vi "tsc-Change Theme Edit--dialog.vi"(8 "error in":errorcluster, 11 "VI Refnum":refnum<vi>) -> (0 "error out":errorcluster)   [LabVIEW 2021]
doc: "Show this VI and let user define a new path/theme to apply to the VI.\n\n->Will be invoked with Quick Drop as a way to easily change the theme quickly during edit mode\n\n<b>Code Developed By:</b>\nTechnology Service Corporation\n1983 S Liberty Drive\nBloomington, IN 47403\nPhone: 812 558-7100\nwww.tsc.com/atcs\n\nDeveloper:\nDaniel Coons"
uses:
  Material Theme/Material Theme.lvclass
  user32.dll
panel:
  out "header":bool
  in  "Done":bool
  in  "Theme":u16(ring) items=["Light Theme", "Light Medium Contrast", "Light High Contrast", "Dark Theme", "Dark Medium Contrast", "Dark High Constrast"]
  in  "file path":path
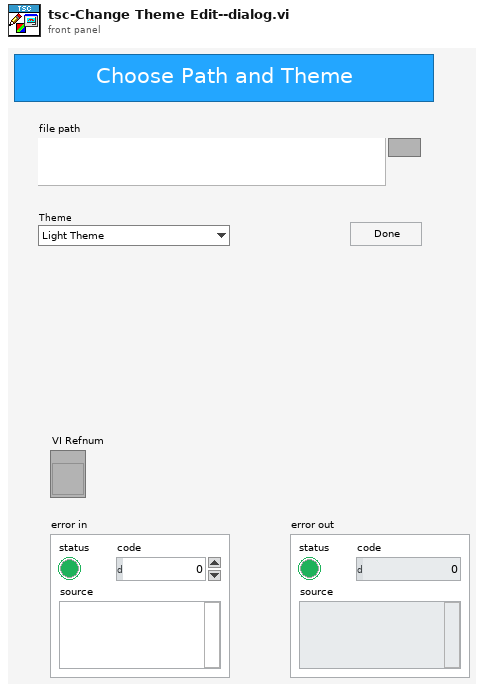
[diagram p1: front panel]
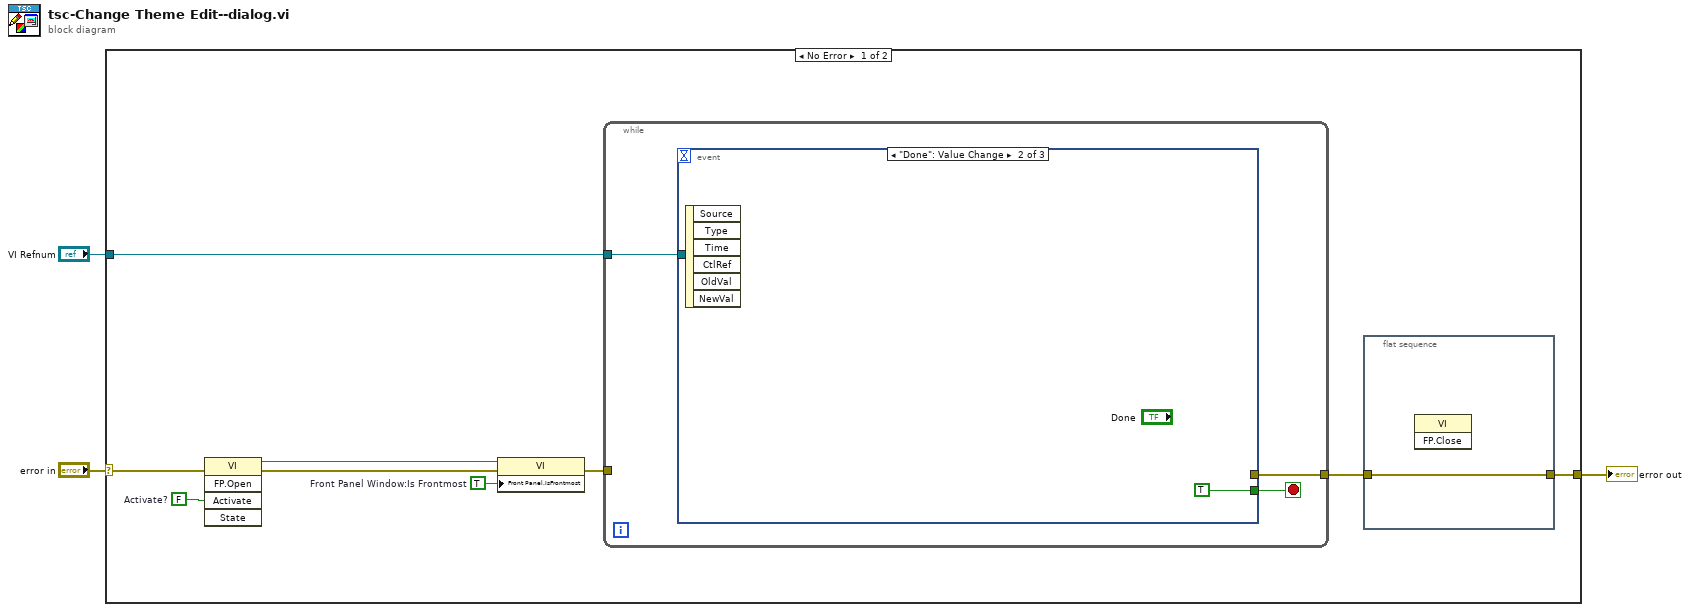
[diagram p0: block diagram]
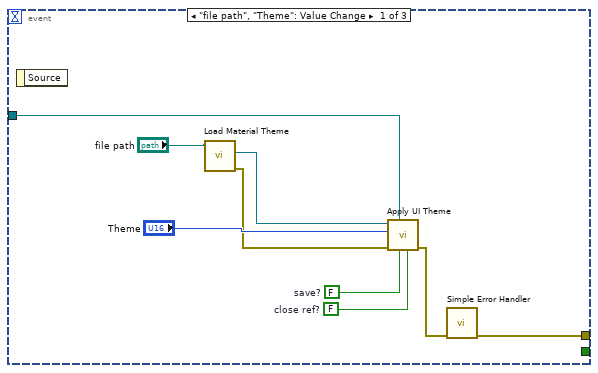
[diagram p2: hidden frame]
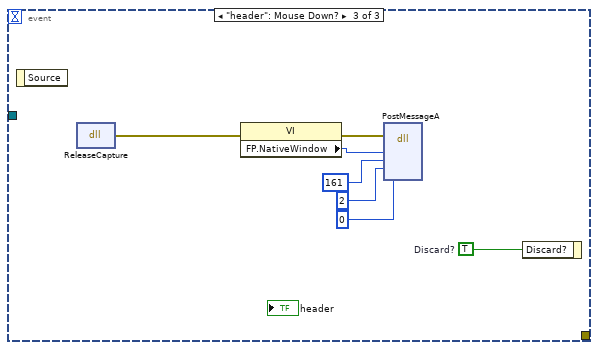
[diagram p3: hidden frame]
diagram:
  n1 = case shown="No Error" "error in" {
    selector: "error in" -> [w11 w34]
    tunnel: "VI Refnum" -> [w12 _]
    tunnel: [w7 w34] -> w2
    frame No Error {
      w4 = TRUE  # Front Panel Window:Is Frontmost
      w9 = FALSE  # Activate?
      n2 = invoke class="VI" method="FP.Open"(error in=w11, "Activate"=w9) -> (reference out=w5:refnum<vi>, error out=w10:errorcluster)  [unwired: 3 in, 3 out]
      n3 = property class="VI"(reference=w5, error in=w10, "Front Panel.IsFrontmost"=w4) -> (error out=w6:errorcluster)  [unwired: 1 out]
      n4 = while {
        tunnel: w12 -> [w16]
        tunnel: w6 -> [_]
        tunnel: [w15] -> w8
        stop <- w14 stop-if-true
        n5 = event shown="[1] \"Done\": Value Change" {
          selector: _ -> [_ _ _]
          dyn-events: _ -> [_ _ _]
          timeout: _ -> [_ _ _]
          tunnel: w16 -> [w22 _ _]
          tunnel: [w19 _ _] -> w15
          tunnel: [_ TRUE _] -> w14
          event "file path", "Theme": Value Change {
            w17 = FALSE  # save?
            w18 = FALSE  # close ref?
            n6 = event-data() -> ()  [unwired: 1 in, 1 out]
            n7 = call "Load Material Theme.vi"("file path (use dialog)"="file path") -> ("error out"=w21:errorcluster, "Theme"=w24:refnum<class "Material Theme.lvclass">)  [unwired: 9 in]
            n8 = call "Apply UI Theme.vi"("close ref?"=w18, "save?"=w17, "VI Refnum"=w22, "error in (no error)"=w21, "Theme"="Theme", "Material Theme in"=w24) -> ("error out"=w20:errorcluster)  [unwired: 4 in, 1 out]
            n9 = call <vilib>:"Simple Error Handler.vi"("error in (no error)"=w20) -> ("error out"=w19:errorcluster)  [unwired: 4 in, 4 out]
          }
          event "Done": Value Change {
            n10 = event-data() -> ()  [unwired: 1 in, 6 out]
          }
          event "header": Mouse Down? {
            w33 = TRUE  # Discard?
            n11 = event-data() -> ()  [unwired: 1 in, 1 out]
            n12 = dll-call lib="user32.dll" fn="ReleaseCapture"() -> (error out=w29:errorcluster)  [unwired: 4 in, 1 out]
            n13 = property class="VI"(error in=w29) -> (error out=w28:errorcluster, "FP.NativeWindow"=w27:u64)  [unwired: 1 in, 1 out]
            n14 = dll-call lib="user32.dll" fn="PostMessageA"(error in=w28, "hWnd"=w27, "Msg"=161, "wParam"=2, "lParam"=0) -> ()  [unwired: 7 in, 2 out]
            n15 = event-data("Discard?"=w33) -> ()  [unwired: 1 in, 1 out]
          }
        }
      }
      n16 = flat-sequence {
        tunnel: w8 -> [w13]
        tunnel: [w13] -> w7
        frame #0 {
          n17 = invoke class="VI" method="FP.Close"() -> ()  [unwired: 3 in, 3 out]
        }
      }
    }
    frame Error {
    }
  }
  "error out" <- w2
